vi "624 Fast CAN Talon SRX Send.vi"(10 "Send This Data":T1={"Output"=0.0, "Control Mode"=enum."Percent VBus", "Brake-Mode Override"=enum."No Override", "Reverse Feedback Sensor"=FALSE, "Reverse Closed-Loop Output"=FALSE, "Override Limits"=FALSE, "Forward Limit Enabled"=FALSE, "Reverse Limit Enabled"=FALSE, "Feedback Select"=0, "Profile Select"=0, "Master To Follow"=0, "Throttle Ramp Rate"=0, "Disabled"=FALSE, "Encoder Codes Per Rev"=0, "Num Pot Turns"=0, "Control Frame Rate Ms"=10, "Use Control5 If Supported"=TRUE, "Enable Frame Rate Ms"=10, "Motion Profile Flow Control"=0, "Motion Profile Control Frame Rate"=10, "Talon SRX Motion Profile Trajectory Point"={"Duration Ms"=0, "Velocity"=0.0, "Position"=0.0, "Profile Slot Select"=0, "Is Last"=FALSE, "Velocity Only"=FALSE, "Zero Position"=FALSE, "Compress Code"=0, "Same Velocity"=0, "Delta Position"=0, "Count"=0}} {"Feedback Select" items=["Digital Quadrature Encoder"=0, "Analog Pot"=2, "Analog Encoder"=3, "Count on Quad-A (Rising-Edge)"=4, "Count on Quad-A (Falling-Edge)"=5, "Position is Pulse-Width"=8, "CTR Magnetic Enc (Relative)"=6, "CTR Magnetic Enc (Absolute)"=7]}, 11 "CAN.Device Number":u8) -> (0 "error out":errorcluster, 3 "Device ID Out":u8)   [LabVIEW 2015]
uses:
  <vilib>/Rock Robotics/WPI/CAN/TalonSRX/WPI_CANTalonSRX_GlobalControl.ctl
  <vilib>/Rock Robotics/WPI/CAN/TalonSRX/WPI_CANTalonSRX_APIControlMode.ctl
  <vilib>/Rock Robotics/WPI/CAN/TalonSRX/WPI_CANTalonSRX_BrakeOverride.ctl
  <vilib>/Rock Robotics/WPI/CAN/TalonSRX/WPI_CANTalonSRX_FeedbackSelect.ctl
  <vilib>/Rock Robotics/WPI/CAN/TalonSRX/WPI_CANTalonSRX_MotionProfileTrajectoryPt.ctl
  <vilib>/Rock Robotics/WPI/CAN/TalonSRX/WPI_CANTalonSRX_ControlMode.ctl
  <vilib>/Rock Robotics/WPI/CAN/TalonSRX/WPI_CANTalonSRX_MessageIDs.ctl
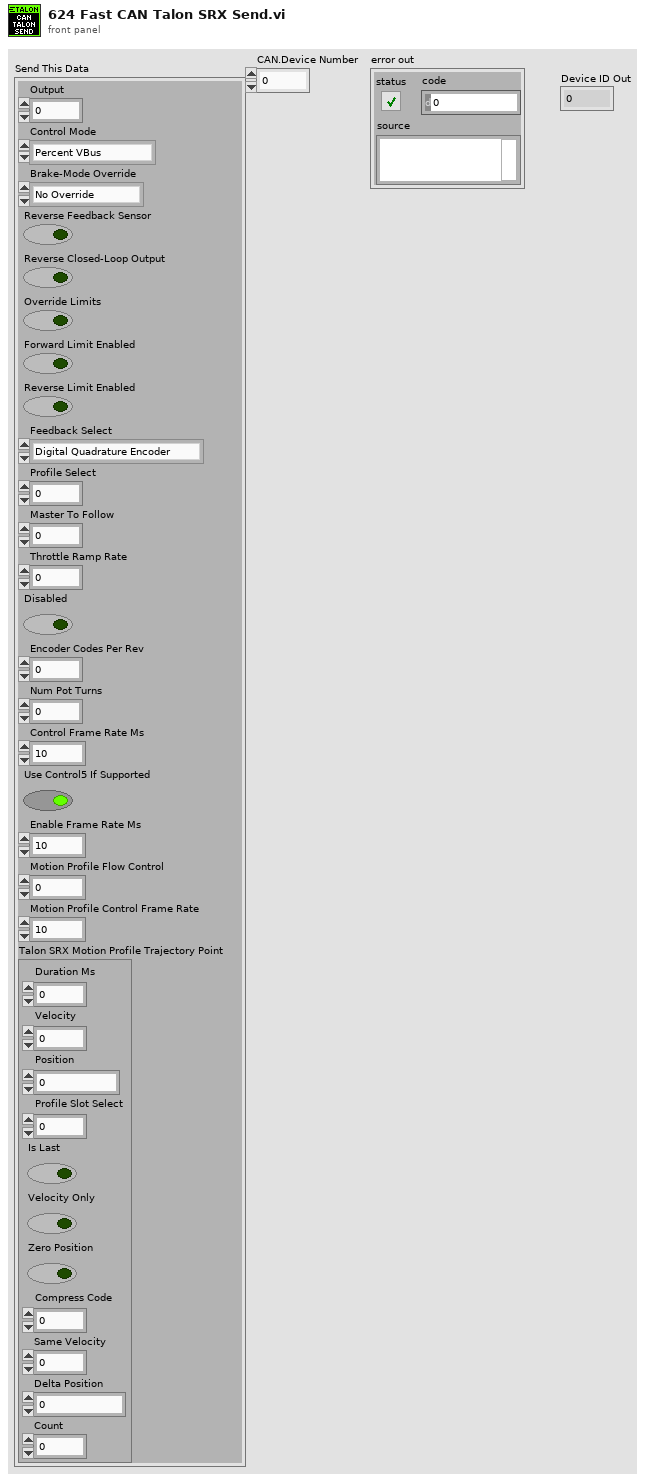
[diagram p1: front panel]
types:
  T1 = typedef "WPI_CANTalonSRX_GlobalControl.ctl" = cluster{"Output":dbl, "Control Mode":T2, "Brake-Mode Override":T3, "Reverse Feedback Sensor":bool, "Reverse Closed-Loop Output":bool, "Override Limits":bool, "Forward Limit Enabled":bool, "Reverse Limit Enabled":bool, "Feedback Select":T4, "Profile Select":u8, "Master To Follow":u8, "Throttle Ramp Rate":u8, "Disabled":bool, "Encoder Codes Per Rev":u32, "Num Pot Turns":u32, "Control Frame Rate Ms":u8, "Use Control5 If Supported":bool, "Enable Frame Rate Ms":u8, "Motion Profile Flow Control":u8, "Motion Profile Control Frame Rate":u8, "Talon SRX Motion Profile Trajectory Point":T5}
  T2 = typedef "WPI_CANTalonSRX_APIControlMode.ctl" = enum8{"Percent VBus", "Speed", "Position", "Slave", "Unchanged / Invalid", "Voltage Compensation", "Current", "Motion Profile"}
  T3 = typedef "WPI_CANTalonSRX_BrakeOverride.ctl" = enum8{"No Override", "Override to Coast", "Override to Brake"}
  T4 = typedef "WPI_CANTalonSRX_FeedbackSelect.ctl" = u8
  T5 = typedef "WPI_CANTalonSRX_MotionProfileTrajectoryPt.ctl" = cluster{"Duration Ms":u8, "Velocity":dbl, "Position":dbl, "Profile Slot Select":u8, "Is Last":bool, "Velocity Only":bool, "Zero Position":bool, "Compress Code":u8, "Same Velocity":i32, "Delta Position":i32, "Count":u8}
  T6 = typedef "WPI_CANTalonSRX_MessageIDs.ctl" = u32
  T7 = typedef "WPI_CANTalonSRX_ControlMode.ctl" = enum16{"Throttle (Duty-Cycle)", "Position Closed-Loop", "Velocity Closed-Loop", "Current Closed-Loop", "Voltage Compensation", "Slave Follower", "Motion Profile"}
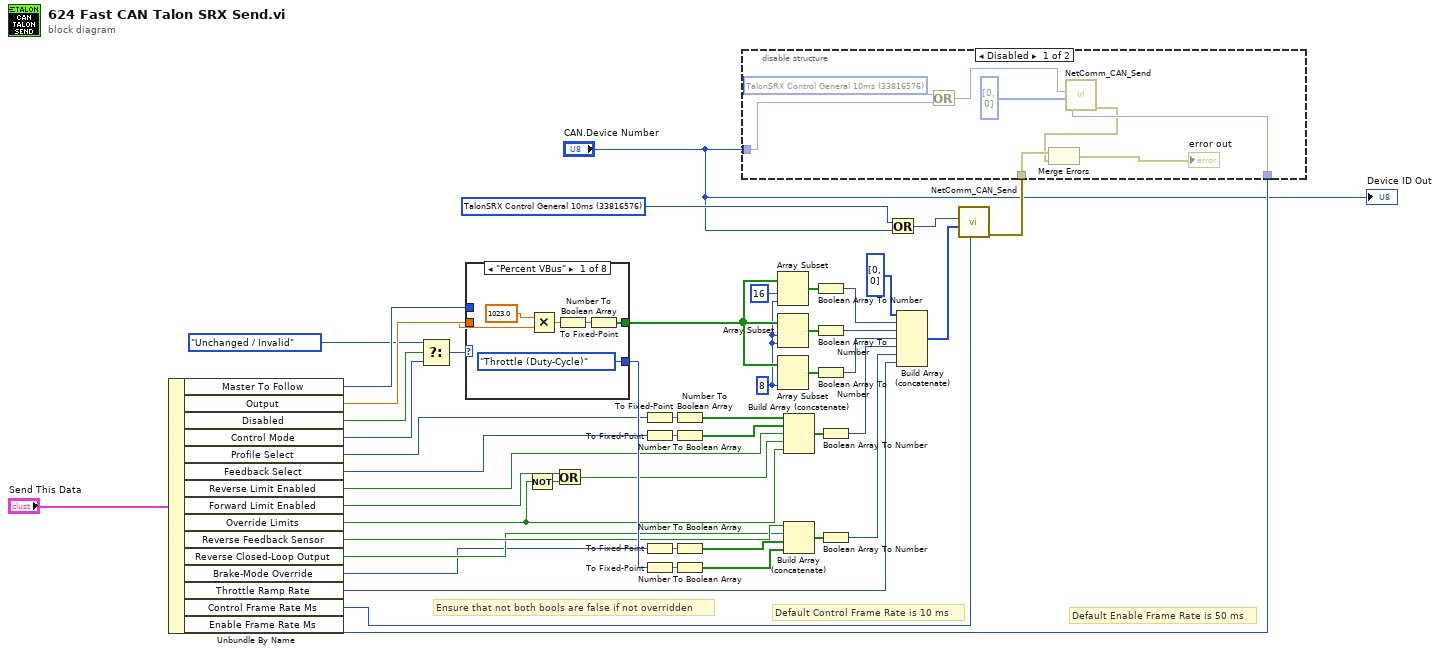
[diagram p0: block diagram]
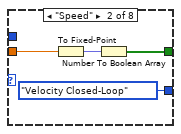
[diagram p3: hidden frame]
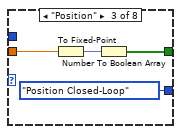
[diagram p4: hidden frame]
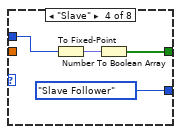
[diagram p5: hidden frame]
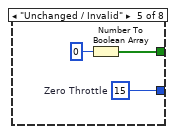
[diagram p6: hidden frame]
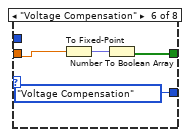
[diagram p7: hidden frame]
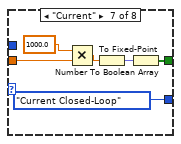
[diagram p8: hidden frame]
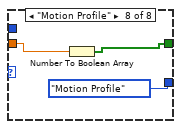
[diagram p9: hidden frame]
diagram:
  w2 = T6 33816576 items=["TalonSRX Control General 10ms"=33816576, "TalonSRX Control Rates Slow"=33816640, "TalonSRX Control ClearFlags Slow"=33816704, "TalonSRX Status General 10ms"=33821696, "TalonSRX Status Feedback 20ms"=33821760, "TalonSRX Status Enc 100ms"=33821824, "TalonSRX Status AinTempVbat 100ms"=33821888, "TalonSRX Status Startup Once"=33821952, "TalonSRX Status Debug"=33822080, "TalonSRX Config SetGainsSlot0 A"=33823808, "TalonSRX Config SetGainsSlot0 B"=33823872, "TalonSRX Config SetGainsSlot1 A"=33823936, "TalonSRX Config SetGainsSlot1 B"=33824000, "TalonSRX Config SetSoftLimits"=33824064, "TalonSRX Config WebControl"=33824128, "TalonSRX Param Request"=33822720, "TalonSRX Param Response"=33822784, "TalonSRX Param Set"=33822848]
  w34 = 8 ("length")
  # "Default Enable Frame Rate is 50 ms"
  # "Default Control Frame Rate is 10 ms"
  # "Ensure that not both bools are false if not overridden"
  n1 = Unbundle By Name("Send This Data") -> ("Master To Follow"=w13:u8, "Output"=w46:dbl, "Disabled"=w9:bool, "Control Mode"=w15:T2, "Profile Select"=w20:u8, "Feedback Select"=w19:T4, "Reverse Limit Enabled"=w23:bool, "Forward Limit Enabled"=w24:bool, "Override Limits"=w21:bool, "Reverse Feedback Sensor"=w18:bool, "Reverse Closed-Loop Output"=w17:bool, "Brake-Mode Override"=w16:T3, "Throttle Ramp Rate"=w12:u8, "Control Frame Rate Ms"=w7:u8, "Enable Frame Rate Ms"=w6:u8)
  n2 = Select(t=WPI_CANTalonSRX_APIControlMode."Unchanged / Invalid", s=w9, f=w15) -> (s? t:f=w10:T2)
  n3 = case shown="\"Percent VBus\"" w10 {
    tunnel: w46 -> [w54 w58 w62 _ _ w70 w76 w80]
    tunnel: [WPI_CANTalonSRX_ControlMode."Throttle (Duty-Cycle)" WPI_CANTalonSRX_ControlMode."Velocity Closed-Loop" WPI_CANTalonSRX_ControlMode."Position Closed-Loop" WPI_CANTalonSRX_ControlMode."Slave Follower" w67 WPI_CANTalonSRX_ControlMode."Voltage Compensation" WPI_CANTalonSRX_ControlMode."Current Closed-Loop" WPI_CANTalonSRX_ControlMode."Motion Profile"] -> w40
    tunnel: [w52 w56 w60 w65 w69 w71 w78 w82] -> w35
    tunnel: w13 -> [_ _ _ w63 _ _ _ _]
    frame "Percent VBus" {
      n4 = Multiply(x=1023.0 ("y"), y=w54) -> (x*y=w50:dbl)
      n5 = To Fixed-Point(number=w50) -> (fixed-point=w49:fxp<+/-,24,24>)  [unwired: 1 in]
      n6 = Number To Boolean Array(number=w49) -> (Boolean array=w52:bool[])
    }
    frame "Speed" {
      n7 = To Fixed-Point(number=w58) -> (fixed-point=w55:fxp<+/-,24,24>)  [unwired: 1 in]
      n8 = Number To Boolean Array(number=w55) -> (Boolean array=w56:bool[])
    }
    frame "Position" {
      n9 = To Fixed-Point(number=w62) -> (fixed-point=w59:fxp<+/-,24,24>)  [unwired: 1 in]
      n10 = Number To Boolean Array(number=w59) -> (Boolean array=w60:bool[])
    }
    frame "Slave" {
      n11 = To Fixed-Point(number=w63) -> (fixed-point=w64:fxp<+,6,6>)  [unwired: 1 in]
      n12 = Number To Boolean Array(number=w64) -> (Boolean array=w65:bool[])
    }
    frame "Unchanged / Invalid" {
      w67 = 15  # Zero Throttle
      n13 = Number To Boolean Array(number=0 ("index")) -> (Boolean array=w69:bool[])
    }
    frame "Voltage Compensation" {
      n14 = To Fixed-Point(number=w70) -> (fixed-point=w72:fxp<+/-,24,16>)  [unwired: 1 in]
      n15 = Number To Boolean Array(number=w72) -> (Boolean array=w71:bool[])
    }
    frame "Current" {
      n16 = Multiply(x=1000.0, y=w76) -> (x*y=w74:dbl)
      n17 = To Fixed-Point(number=w74) -> (fixed-point=w79:fxp<+/-,24,24>)  [unwired: 1 in]
      n18 = Number To Boolean Array(number=w79) -> (Boolean array=w78:bool[])
    }
    frame "Motion Profile" {
      n19 = Number To Boolean Array(number=w80) -> (Boolean array=w82:bool[])
    }
  }
  n20 = Not(x=w21) -> (.not. x?=w14:bool)
  n21 = Or(x=w24, y=w14) -> (x .or. y?=w22:bool)
  n22 = To Fixed-Point(number=w20) -> (fixed-point=w5:fxp<+,1,1>)  [unwired: 1 in]
  n23 = To Fixed-Point(number=w19) -> (fixed-point=w32:fxp<+,4,4>)  [unwired: 1 in]
  n24 = To Fixed-Point(number=w16) -> (fixed-point=w28:fxp<+,2,2>)  [unwired: 1 in]
  n25 = To Fixed-Point(number=w40) -> (fixed-point=w41:fxp<+,4,4>)  [unwired: 1 in]
  n26 = Number To Boolean Array(number=w5) -> (Boolean array=w25:bool[])
  n27 = Number To Boolean Array(number=w32) -> (Boolean array=w31:bool[])
  n28 = Number To Boolean Array(number=w28) -> (Boolean array=w27:bool[])
  n29 = Number To Boolean Array(number=w41) -> (Boolean array=w26:bool[])
  n30 = Array Subset(array=w35, index=16, length=w34) -> (w36:bool[])
  n31 = Array Subset(array=w35, index=w34, length=w34) -> (w38:bool[])
  n32 = Array Subset(array=w35, length=w34) -> (w37:bool[])  [unwired: 1 in]
  n33 = Build Array (concatenate)(w25, w31, w23, w22, w21) -> (w30:bool[])
  n34 = Build Array (concatenate)(w18, w17, w27, w26) -> (w42:bool[])
  n35 = Boolean Array To Number(Boolean array=w36) -> (number=w39:u32)
  n36 = Boolean Array To Number(Boolean array=w38) -> (number=w44:u32)
  n37 = Boolean Array To Number(Boolean array=w37) -> (number=w43:u32)
  n38 = Boolean Array To Number(Boolean array=w30) -> (number=w29:u32)
  n39 = Boolean Array To Number(Boolean array=w42) -> (number=w45:u32)
  n40 = Or(x=w2, y="CAN.Device Number") -> (x .or. y?=w3:T6)
  n41 = Build Array (concatenate)(u8[] [0, 0] ("Token Space"), w39, w44, w43, w29, w45, w12) -> (w48:u32[])
  n42 = call <vilib>:"NetComm_CAN_Send.vi"("Period (ms)"=w7, "Data"=w48, "Message ID"=w3) -> ("error out"=w11:errorcluster)  [unwired: 8 in]
  n43 = disable-structure shown="Disabled" {
    disable-tunnel: w11 -> [w90 _]
    disable-tunnel: w6 -> [w88 _]
    disable-tunnel: "CAN.Device Number" -> [w84 _]
    frame Disabled {
      w86 = T6 33816576 items=["TalonSRX Control General 10ms"=33816576, "TalonSRX Control Rates Slow"=33816640, "TalonSRX Control ClearFlags Slow"=33816704, "TalonSRX Status General 10ms"=33821696, "TalonSRX Status Feedback 20ms"=33821760, "TalonSRX Status Enc 100ms"=33821824, "TalonSRX Status AinTempVbat 100ms"=33821888, "TalonSRX Status Startup Once"=33821952, "TalonSRX Status Debug"=33822080, "TalonSRX Config SetGainsSlot0 A"=33823808, "TalonSRX Config SetGainsSlot0 B"=33823872, "TalonSRX Config SetGainsSlot1 A"=33823936, "TalonSRX Config SetGainsSlot1 B"=33824000, "TalonSRX Config SetSoftLimits"=33824064, "TalonSRX Config WebControl"=33824128, "TalonSRX Param Request"=33822720, "TalonSRX Param Response"=33822784, "TalonSRX Param Set"=33822848]
      n44 = Or(x=w86, y=w84) -> (x .or. y?=w87:T6)
      n45 = call <vilib>:"NetComm_CAN_Send.vi"("Period (ms)"=w88, "Data"=u8[] [0, 0] ("Token Space"), "Message ID"=w87) -> ("error out"=w83:errorcluster)  [unwired: 8 in]
      n46 = Merge Errors(w90, w83) -> (→"error out":errorcluster)
    }
    frame Enabled {
    }
  }
  "Device ID Out" <- "CAN.Device Number"
